vi "set_params.vi"(8 "error in (no error)":errorcluster caption="entrée d'erreur (pas d'erreur)", 11 "AffinityPropagation.lvclass 2":refnum<class "AffinityPropagation.lvclass">) -> (0 "error out":errorcluster caption="sortie d'erreur", 3 "AffinityPropagation.lvclass":refnum<class "AffinityPropagation.lvclass">)   [LabVIEW 2020, in "AffinityPropagation.lvclass"]
uses:
  AffinityPropagation.lvclass
  AffinityPropagation.lvclass/AffinityPropagation.ctl
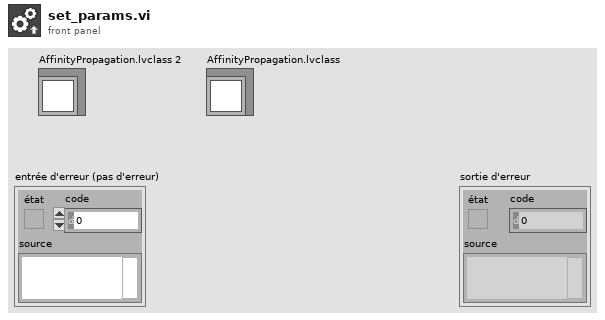
[diagram p1: front panel]
types:
  T1 = typedef "affinity_propagation_params.ctl" = cluster{"damping":dbl, "max_iter":i32, "convergence_iter":i32, "copy":bool, "preference":cluster{"preference_type":string, "preference_list":dbl[], "preference_float":dbl}, "affinity":string, "verbose":bool, "random_state":i32}
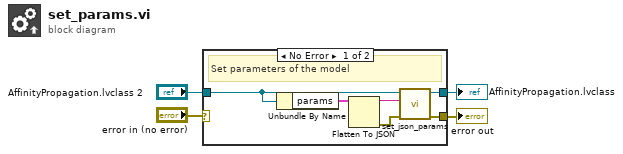
[diagram p0: block diagram]
diagram:
  n1 = case shown="No Error" "error in (no error)" {
    selector: "error in (no error)" -> [_ w12]
    tunnel: [w7 w12] -> w3
    tunnel: [w8 w11] -> w1
    tunnel: "AffinityPropagation.lvclass 2" -> [w5 w11]
    frame No Error {
      # "Set parameters of the model"
      n2 = Unbundle By Name(w5) -> ("params"=w10:T1)
      n3 = Flatten To JSON(anything=w10) -> (JSON string=w9:string, 11:w6:errorcluster)  [unwired: 2 in]
      n4 = call-dynamic "set_json_params.vi"("error in (no error)"=w6, "params"=w9, "Model en entrée"=w5) -> ("error out"=w7:errorcluster, "Model en sortie"=w8:refnum<class "AffinityPropagation.lvclass">)  [unwired: 7 in]
    }
    frame Error {
    }
  }
  "error out" <- w3
  "AffinityPropagation.lvclass" <- w1
